vi "Routine.Create.vi"(8 "error in (no error)":errorcluster, 10 "Routine":T1 {"Stop Parameters"."Response"."Byte Order" items=["Little Endian", "Big Endian"]; "Stop Parameters"."Response"."Data Type" items=["Signed", "Unsigned", "IEEE Float"]; "Stop Parameters"."Cmd"."Byte Order" items=["Little Endian", "Big Endian"]; "Stop Parameters"."Cmd"."Data Type" items=["Signed", "Unsigned", "IEEE Float"]; "Request Parameters"."Response"."Byte Order" items=["Little Endian", "Big Endian"]; "Request Parameters"."Response"."Data Type" items=["Signed", "Unsigned", "IEEE Float"]; "Request Parameters"."Cmd"."Byte Order" items=["Little Endian", "Big Endian"]; "Request Parameters"."Cmd"."Data Type" items=["Signed", "Unsigned", "IEEE Float"]; "Start Parameters"."Response"."Byte Order" items=["Little Endian", "Big Endian"]; "Start Parameters"."Response"."Data Type" items=["Signed", "Unsigned", "IEEE Float"]; "Start Parameters"."Cmd"."Byte Order" items=["Little Endian", "Big Endian"]; "Start Parameters"."Cmd"."Data Type" items=["Signed", "Unsigned", "IEEE Float"]}, 11 "Section Ptr":T4 format="%.0x") -> (0 "error out":errorcluster, 3 "Parent Ref out":T4 format="%.0x")   [LabVIEW 2019, in "Diagnostics Addon System Explorer.lvlib"]
uses:
  Diagnostics Addon System Explorer.lvlib
  <vilib>/NI VeriStand/Custom Device API/Custom Device Item Ref.ctl
  Types/Routine.Export.ctl
  Types/CmdResp.Export.ctl
  Addon Shared/Types/Signal.ctl
  Addon Shared/Types/Type.ctl
  Types/FG.Action.ctl
  Addon Shared/SubVIs/Constants.vi
  <vilib>/NI/NI VeriStand Advanced SysDef API/SysDef API/SysDef.Property.Set.vi
  <vilib>/NI/NI VeriStand Advanced SysDef API/_SubVIs/SysDef.Property.Set.U32.vi
  <vilib>/NI VeriStand/Custom Device API/NI VeriStand - Get Item Property.vi
  <vilib>/NI VeriStand/Custom Device API/Get Item Property (U32).vi
  Addon Shared/Diagnostics Addon Shared.lvlib
  <vilib>/NI/NI VeriStand Advanced SysDef API/SysDef API/Advanced System Definition.lvlib
  <vilib>/NI VeriStand/Custom Device API/Custom Device API.lvlib
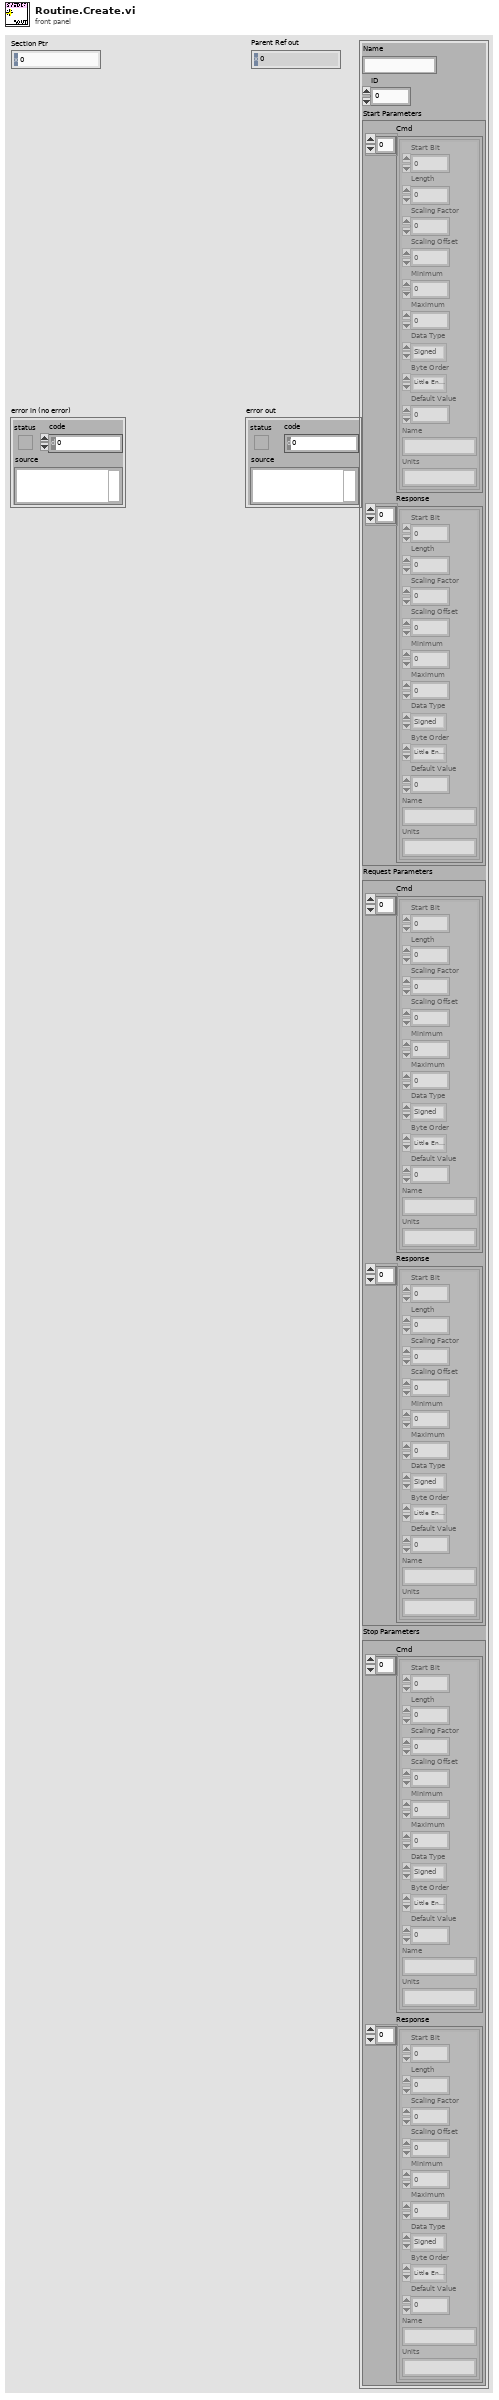
[diagram p1: front panel]
types:
  T1 = typedef "Diagnostics Addon System Explorer.lvlib/Routine.Export.ctl" = cluster{"Name":string, "ID":u16, "Start Parameters":T2, "Request Parameters":T2, "Stop Parameters":T2}
  T2 = typedef "Diagnostics Addon System Explorer.lvlib/CmdResp.Export.ctl" = cluster{"Cmd":T3[], "Response":T3[]}
  T3 = typedef "Diagnostics Addon Shared.lvlib/Signal.ctl" = cluster{"Start Bit":u32, "Length":u32, "Scaling Factor":dbl, "Scaling Offset":dbl, "Minimum":dbl, "Maximum":dbl, "Data Type":u32, "Byte Order":u32, "Default Value":dbl, "Name":string, "Units":string}
  T4 = typedef "Custom Device API.lvlib/Custom Device Item Ref.ctl" = u64
  T5 = typedef "Diagnostics Addon Shared.lvlib/Type.ctl" = enum16{"DID", "CDID", "PID", "CPID", "Read Memory", "Write Memory", "IO Control", "Routine Start", "Routine Request", "Routine Stop", "User Defined", "DTC Control", "Clear DTCs", "Read DTCs", "Start DTCs", "DTC Change Count", "Tester Present", "Unlock ECU", "Reset ECU", "Diag Session Control", "Communication Control", "DPID Control", "Poll Control", "Diag CAN Control"}
  T6 = typedef "Diagnostics Addon System Explorer.lvlib/FG.Action.ctl" = enum16{"Get", "Set"}
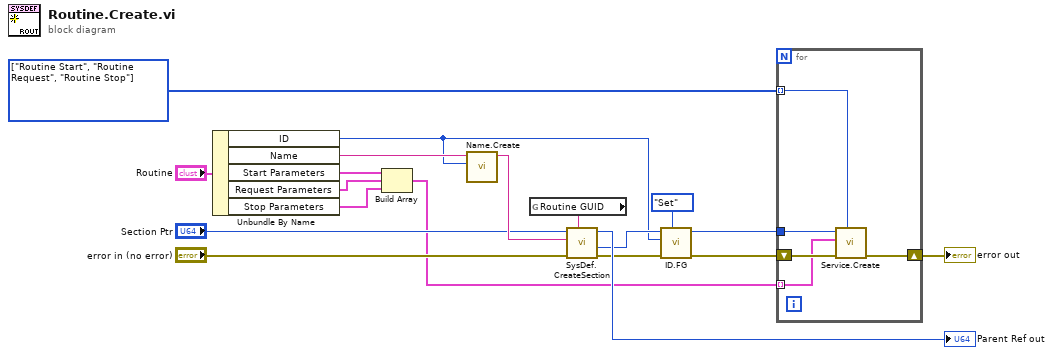
[diagram p0: block diagram]
diagram:
  w5 = T5[] [enum."Routine Start", enum."Routine Request", enum."Routine Stop"] items=["DID", "CDID", "PID", "CPID", "Read Memory", "Write Memory", "IO Control", "Routine Start", "Routine Request", "Routine Stop", "User Defined", "DTC Control", "Clear DTCs", "Read DTCs", "Start DTCs", "DTC Change Count", "Tester Present", "Unlock ECU", "Reset ECU", "Diag Session Control", "Communication Control", "DPID Control", "Poll Control", "Diag CAN Control"]
  n1 = Unbundle By Name("Routine") -> ("ID"=w8:u16, "Name"=w17:string, "Start Parameters"=w4:T2, "Request Parameters"=w3:T2, "Stop Parameters"=w2:T2)
  n2 = Build Array(w4, w3, w2) -> (w1:T2[])
  n3 = call "Name.Create.vi"("PID Number"=w8, "PID Name"=w17) -> ("VS Name"=w19:string)  [unwired: 9 in]
  n4 = global read "Constants.vi" "Routine GUID"() -> (w16:string)
  n5 = call <vilib>:"SysDef.CreateSection.vi"("GUID"=w16, "error in (no error)"="error in (no error)", "Name"=w19, "nodeID"="Section Ptr") -> ("error out"=w10:errorcluster, "New NodeID"=w9:u64, "nodeID out"=→"Parent Ref out":u64)  [unwired: 4 in, 1 out]
  n6 = call "ID.FG.vi"("Action"=FG.Action."Set", "error in (no error)"=w10, "ID"=w8, "Device Item Ref in"=w9) -> ("error out"=w7:errorcluster, "Device Item Ref out"=w6:T4)  [unwired: 5 in, 1 out]
  n7 = for {
    tunnel: w6 -> [w24]
    shift-right: [w22] -> w13
    shift-left: w7 -> [w23]
    tunnel: w5 -> [w21] mode=indexing
    tunnel: w1 -> [w20] mode=indexing
    n8 = call "Service.Create.vi"("Type"=w21, "error in (no error)"=w23, "Variant"=w20, "Section Ptr"=w24) -> ("error out"=w22:errorcluster)  [unwired: 6 in, 1 out]
  }
  "error out" <- w13
